vi "bubble sorting.vi"(2 "value between1~10000":dbl[](array[numeric]), 4 "N numbers":i32) -> ()   [LabVIEW 2014]
panel:
  out "Bubble Sort Waveform bar graph":dbl[](graph)
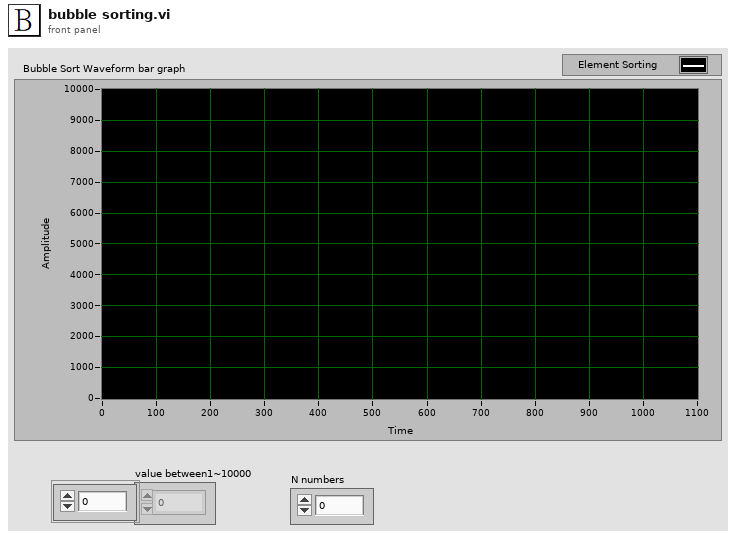
[diagram p1: front panel]
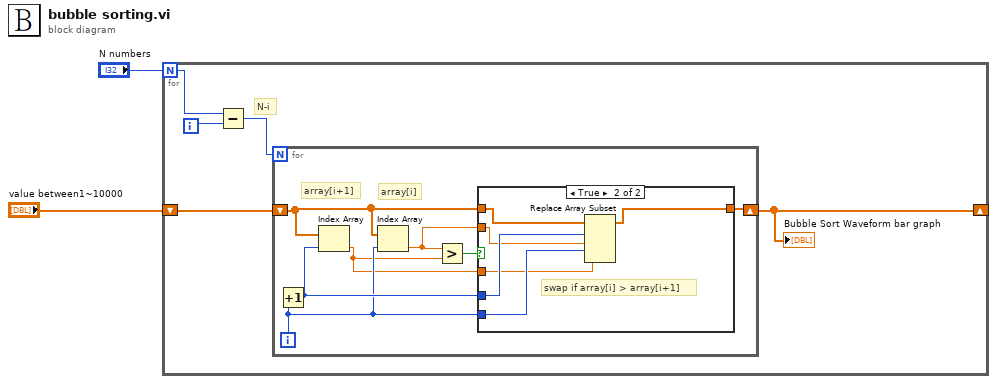
[diagram p0: block diagram]
diagram:
  n1 = for {
    N: "N numbers" -> [w7]
    shift-right: [w3] -> _
    shift-left: "value between1~10000" -> [w4]
    i -> [w6]
    # "N-i"
    n2 = Subtract(x=w7, y=w6) -> (x-y=w5:i32)
    n3 = for {
      N: w5 -> [_]
      shift-right: [w12] -> w3
      shift-left: w4 -> [w14]
      i -> [w10]
      # "array[i]"
      # "array[i+1]"
      n4 = Increment(x=w10) -> (x+1=w11:i32)
      n5 = Index Array(array=w14, index=w11) -> (element=w8:dbl)
      n6 = Index Array(array=w14, index=w10) -> (element=w9:dbl)
      n7 = Greater?(x=w9, y=w8) -> (0:w13:bool)
      n8 = case shown="True" w13 {
        tunnel: w14 -> [w15 w17]
        tunnel: [w15 w16] -> w12
        tunnel: w10 -> [_ w20]
        tunnel: w11 -> [_ w21]
        tunnel: w9 -> [_ w19]
        tunnel: w8 -> [_ w18]
        frame False {
        }
        frame True {
          # "swap if array[i] > array[i+1]"
          n9 = Replace Array Subset(array=w17, new element #1=w19, index #1=w21, new element #2=w18, index #2=w20) -> (w16:dbl[])
        }
      }
    }
    "Bubble Sort Waveform bar graph" <- w3
  }
